vi "DFT_Spectra Global.vi"() -> ()   [LabVIEW 2024, in "DFT_Spectra.lvlib" / "DFT_Spectra.lvclass"]
uses:
  DFT_Spectra.lvclass
panel:
  in  "Block duration":string="Block duration"
  in  "Weighting mode strings":string[](array[string])=["Exponential"]
  in  "Averaging mode strings":string[](array[string])=["No averaging", "RMS averaging", "Peak hold"]
  in  "Window values":u32[](array[ring])=[0, 1, 6, 8] items=["Rectangle"=0, "Hanning"=1, "Hamming"=2, "Blackman-Harris"=3, "Exact Blackman"=4, "Blackman"=5, "Flat Top"=6, "4 Term B-Harris "=7, "7 Term B-Harris"=8, "Low Sidelobe"=9, "Blackman Nuttall"=11, "Triangle"=30, "Bartlett-Hanning"=31, "Bohman"=32, "Parzen"=33, "Welch"=34, "Kaiser"=60, "Dolph-Chebyshev"=61, "Gaussian"=62]
  in  "Weighting mode values":enum16{"Linear", "Exponential"}[](array[ring])=[enum."Exponential"]
  in  "Averaging mode values":T1(array[ring])=[enum."No averaging", enum."RMS averaging", enum."Peak hold"]
  in  "Overlap":string="Overlap"
  in  "Number of averages":string="Number of averages"
  in  "Weighting mode":string="Weighting mode"
  in  "Window Strings":string[](array[string])=["Rectangle", "Hanning", "Flat Top", "7 Term B-Harris"]
  in  "Averaging mode":string="Averaging mode"
  in  "Window":string="Window"
  in  "Show UI":string="Show Frequency Spectra"
  in  "Select Channel":string="Select Channel(s)"
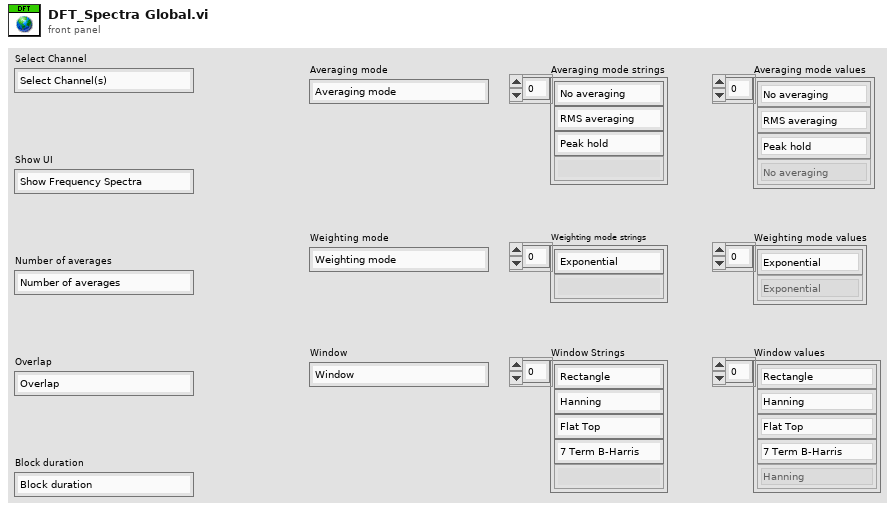
[diagram p1: front panel]
types:
  T1 = enum16{"No averaging", "Vector averaging", "RMS averaging", "Peak hold"}[]
diagram:
